vi "Sub (control and indicator).vi"(1 "Bool Refnum":refnum<vi>, 2 "WFChart Refnum":refnum<vi>) -> ()   [LabVIEW 2013]
doc: "The program uses a Control Reference to give access to a front panel control, to a subVI. The main program calls the subVI. The subVI then writes a random number to the Waveform Chart in the front panel of the main VI. It reads the value from the Boolean control in the main VI front panel to terminate execution of the while loop. The Control References were created by right-clicking on the waveform chart or Boolean terminal and selecting Create > Reference. The Waveform Chart Refnum in the subVI can be created in two ways.\n1. Dragging the Control Reference from the Block Diagram of the Main VI to the Front Panel of the subVI.\n2. Place a Control Refnum of the Front Panel of the subVI by selecting Controls > Refnum > Control Refnum. Then select a Waveform Chart form the Controls palette and drop it inside the Control Refnum Container.\n\nThe Boolean Refnum was created in a similar manner."
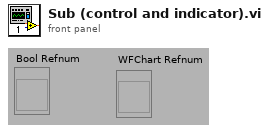
[diagram p1: front panel]
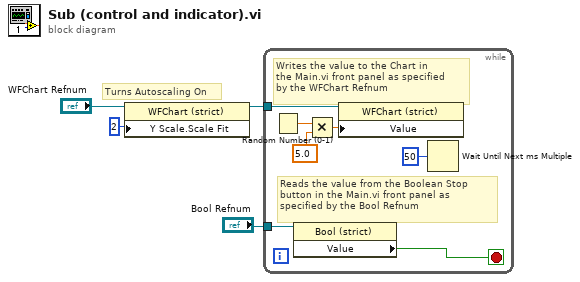
[diagram p0: block diagram]
diagram:
  # "Turns Autoscaling On"
  n1 = property class="WFChart (strict)"(reference="WFChart Refnum", "Y Scale.Scale Fit"=u8 2) -> (reference out=w3:refnum<vi>)  [unwired: 1 in, 1 out]
  n2 = while {
    tunnel: w3 -> [w10]
    tunnel: "Bool Refnum" -> [w5]
    stop <- w6 stop-if-true
    # "Reads the value from the Boolean Stop\nbutton in the Main.vi front panel as\nspecified by the Bool Refnum"
    # "Writes the value to the Chart in\nthe Main.vi front panel as specified\nby the WFChart Refnum"
    n3 = Random Number (0-1)() -> (number: 0 to 1=w9:dbl)
    n4 = property class="Bool (strict)"(reference=w5) -> ("Value"=w6:bool)  [unwired: 1 in, 2 out]
    n5 = Multiply(x=w9, y=5.0) -> (x*y=w7:dbl)
    n6 = property class="WFChart (strict)"(reference=w10, "Value"=w7) -> ()  [unwired: 1 in, 2 out]
    n7 = Wait Until Next ms Multiple(millisecond multiple=u32 50) -> ()  [unwired: 1 out]
  }
